vi "SUB_RF_Result_StringChk.vi"(3 "Input String":string) -> (1 "Output String":string)   [LabVIEW 2011]
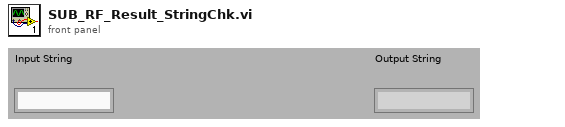
[diagram p1: front panel]
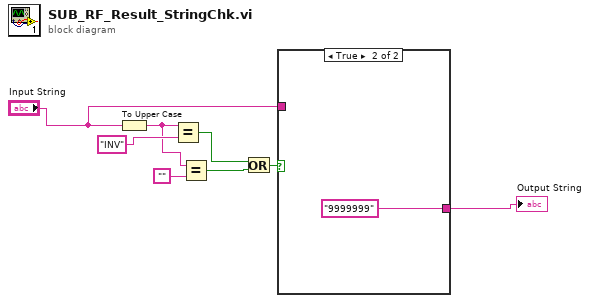
[diagram p0: block diagram]
diagram:
  n1 = To Upper Case(1:"Input String") -> (0:w7:string)
  n2 = Equal?(x=w7, y="INV") -> (x = y?=w4:bool)
  n3 = Equal?(x=w7, y="") -> (x = y?=w3:bool)
  n4 = Or(x=w4, y=w3) -> (x .or. y?=w5:bool)
  n5 = case shown="True" w5 {
    tunnel: [w9 "9999999"] -> w2
    tunnel: "Input String" -> [w9 _]
    frame False {
    }
    frame True {
    }
  }
  "Output String" <- w2
